vi "Move piezo slow.vi"(7 "error in (no error)":errorcluster, 8 "MOVE TO [MICRON]":dbl=1.0 format="%0.2f", 9 "notifier out":refnum<notifier>, 10 "Cluster":T1={"physical channels"="Dev5/ao0", "MAX   VOLTAGE"=10.0, "MIN   VOLTAGE"=0.0}) -> (0 "error out":errorcluster, 3 "Cluster 2":T1={"physical channels"="Dev5/ao0", "MAX   VOLTAGE"=10.0, "MIN   VOLTAGE"=0.0})   [LabVIEW 2013]
uses:
  Piezo/Piezo display.ctl
  Untitled Project 3 Andrea/piezo new/Hardware Configuration Piezo out.ctl
  <vilib>/Analysis/1siggen.llb/Ramp Pattern by Samples.vi
  <vilib>/DAQmx/write.llb/DAQmx Write (Analog DBL 1Chan 1Samp).vi
  <vilib>/DAQmx/create/channels.llb/DAQmx Create Channel (AO-Voltage-Basic).vi
  <vilib>/DAQmx/miscellaneous.llb/DAQmx Fill In Error Info.vi
  <vilib>/Analysis/NI_AALBase.lvlib
  Piezo/Piezo.lvlib
panel:
  out "PiezoPosition":sgl
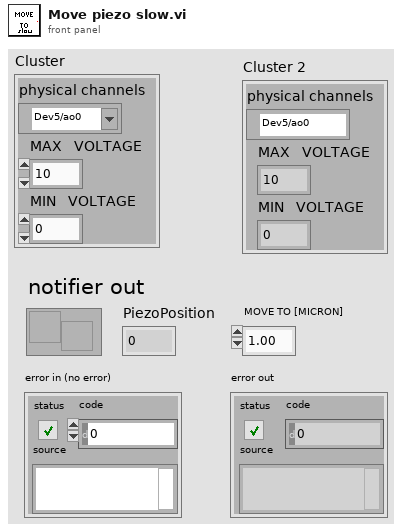
[diagram p1: front panel]
types:
  T1 = typedef "Hardware Configuration Piezo out.ctl" = cluster{"physical channels":tag, "MAX   VOLTAGE":dbl, "MIN   VOLTAGE":dbl}
  T2 = typedef "Piezo.lvlib/Piezo display.ctl" = cluster{"PiezoPosition":sgl, "Counter Time":i32}
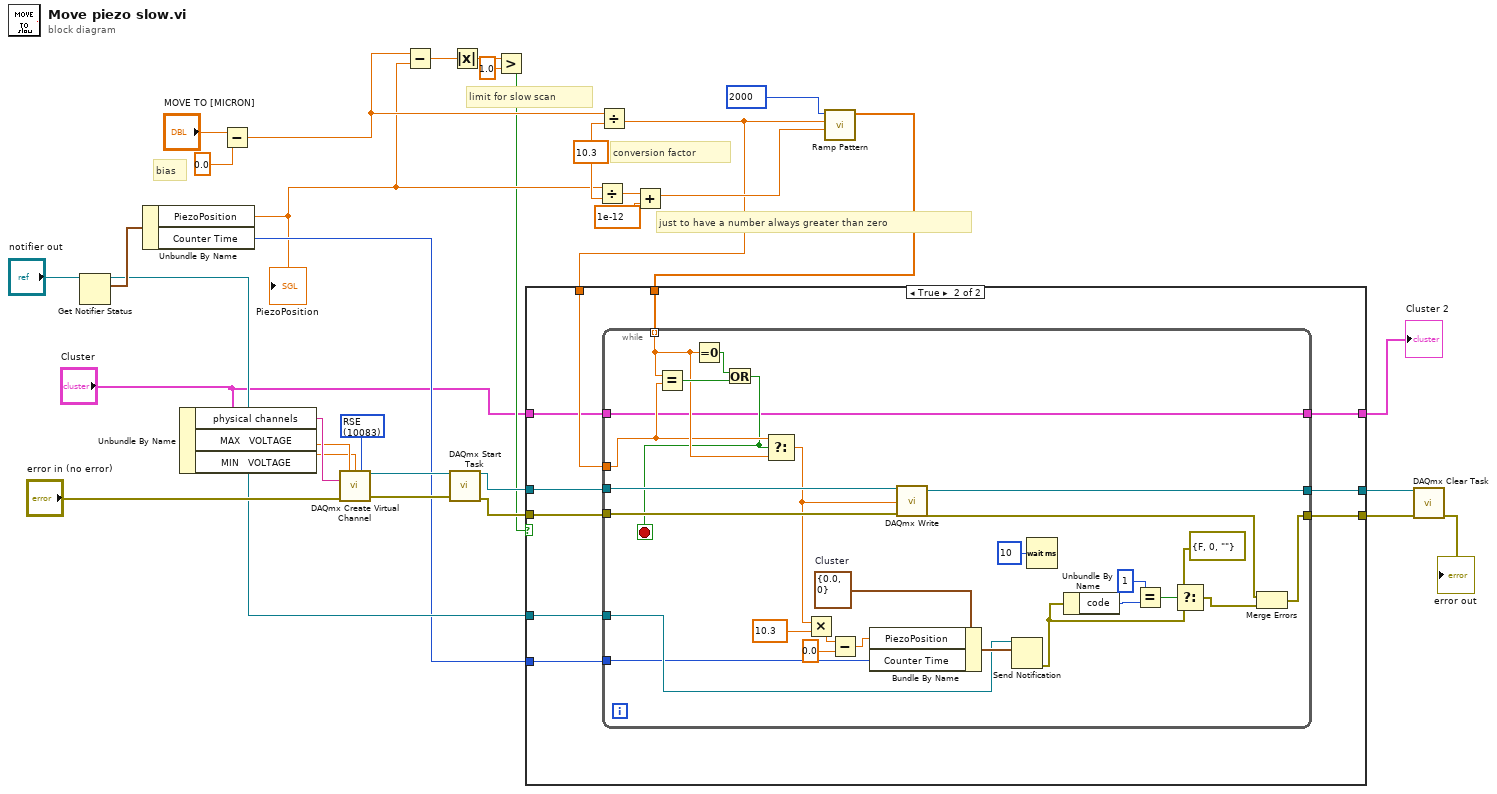
[diagram p0: block diagram]
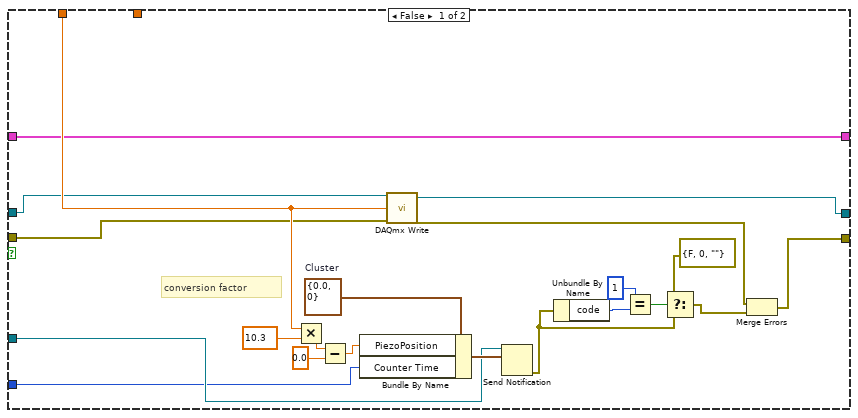
[diagram p2: hidden frame]
diagram:
  w25 = 10083 items=["Default"=-1, "RSE"=10083, "Differential"=10106, "Pseudodifferential"=12529] ("output terminal configuration")
  w30 = 10.3
  # "limit for slow scan"
  # "just to have a number always greater than zero"
  # "bias"
  # "conversion factor"
  n1 = Get Notifier Status(notifier="notifier out") -> (notifier out=w13:refnum<notifier>, current notification=w26:T2)  [unwired: 1 in, 3 out]
  n2 = Unbundle By Name(w26) -> ("PiezoPosition"=w4:sgl, "Counter Time"=w12:i32)
  "PiezoPosition" <- w4
  n3 = Unbundle By Name("Cluster") -> ("physical channels"=w22:tag, "MAX   VOLTAGE"=w21:dbl, "MIN   VOLTAGE"=w20:dbl)
  n4 = Subtract(x="MOVE TO [MICRON]", y=0.0) -> (x-y=w5:dbl)
  n5 = call-poly <vilib>:"DAQmx Create Virtual Channel.vi"("maximum value"=w21, "minimum value"=w20, "output terminal configuration"=w25, "physical channels"=w22, "error in"="error in (no error)") -> ("task out"=w24:refnum<k21>, "error out"=w23:errorcluster)  [unwired: 9 in]
  n6 = Subtract(x=w5, y=w4) -> (x-y=w8:dbl)
  n7 = call <vilib>:"DAQmx Start Task.vi"("task/channels in"=w24, "error in"=w23) -> ("task out"=w16:refnum<k21>, "error out"=w15:errorcluster)  [unwired: 12 in]
  n8 = Absolute Value(x=w8) -> (abs(x)=w7:dbl)
  n9 = Greater?(x=w7, y=1.0) -> (0:w3:bool)
  n10 = Divide(x=w4, y=w30) -> (x/y=w31:dbl)
  n11 = Divide(x=w5, y=w30) -> (x/y=w28:dbl)
  n12 = Add(x=w31, y=1e-12) -> (x+y=w32:dbl)
  n13 = call-poly <vilib>:"Ramp Pattern.vi"("start"=w32, "end"=w28, "samples"=2000) -> ("Ramp Pattern"=w29:dbl[])  [unwired: 7 in, 1 out]
  n14 = case shown="True" w3 {
    tunnel: w29 -> [_ w64]
    tunnel: w28 -> [w41 w63]
    tunnel: [w38 w62] -> w18
    tunnel: [w37 w61] -> w17
    tunnel: w16 -> [w40 w60]
    tunnel: w15 -> [w39 w59]
    tunnel: "Cluster" -> [w34 w58]
    tunnel: [w34 w57] -> w1
    tunnel: w13 -> [w36 w56]
    tunnel: w12 -> [w35 w55]
    frame False {
      w53 = T2 {"PiezoPosition"=0.0, "Counter Time"=0}  # Cluster
      # "conversion factor"
      n15 = Multiply(x=w41, y=10.3) -> (x*y=w43:dbl)
      n16 = Subtract(x=w43, y=0.0) -> (x-y=w44:dbl)
      n17 = Bundle By Name(cluster=w53, "PiezoPosition"=w44, "Counter Time"=w35) -> (w54:T2)
      n18 = call-poly <vilib>:"DAQmx Write.vi"("task/channels in"=w40, "data"=w41, "error in"=w39) -> ("task out"=w38:refnum<k21>, "error out"=w48:errorcluster)  [unwired: 10 in, 1 out]
      n19 = Send Notification(notification=w54, notifier=w36) -> (error out=w47:errorcluster)  [unwired: 1 in, 1 out]
      n20 = Unbundle By Name(w47) -> ("code"=w52:i32)
      n21 = Equal?(x=1, y=w52) -> (x = y?=w50:bool)
      n22 = Select(t=errorcluster {"status"=FALSE, "code"=0, "source"=""} ("error constant"), s=w50, f=w47) -> (s? t:f=w46:errorcluster)
      n23 = Merge Errors(w48, w46) -> (w37:errorcluster)
    }
    frame True {
      n24 = while {
        tunnel: w60 -> [w91]
        tunnel: w59 -> [w90]
        tunnel: [w89] -> w62
        tunnel: [w70] -> w61
        tunnel: w64 -> [w86] mode=indexing
        tunnel: w63 -> [w85]
        tunnel: w58 -> [w82]
        tunnel: [w82] -> w57
        tunnel: w56 -> [w80]
        tunnel: w55 -> [w78]
        stop <- w84 stop-if-true
        w79 = T2 {"PiezoPosition"=0.0, "Counter Time"=0}  # Cluster
        n25 = Equal?(x=w86, y=w85) -> (x = y?=w87:bool)
        n26 = Equal To 0?(x=w86) -> (x = 0?=w88:bool)
        n27 = Or(x=w88, y=w87) -> (x .or. y?=w84:bool)
        n28 = Select(t=w85, s=w84, f=w86) -> (s? t:f=w68:dbl)
        n29 = Multiply(x=w68, y=10.3) -> (x*y=w66:dbl)
        n30 = Subtract(x=w66, y=0.0) -> (x-y=w67:dbl)
        n31 = Bundle By Name(cluster=w79, "PiezoPosition"=w67, "Counter Time"=w78) -> (w81:T2)
        n32 = call-poly <vilib>:"DAQmx Write.vi"("task/channels in"=w91, "data"=w68, "error in"=w90) -> ("task out"=w89:refnum<k21>, "error out"=w73:errorcluster)  [unwired: 10 in, 1 out]
        n33 = Send Notification(notification=w81, notifier=w80) -> (error out=w72:errorcluster)  [unwired: 1 in, 1 out]
        n34 = Wait (ms)(milliseconds to wait=u32 10) -> ()  [unwired: 1 out]
        n35 = Unbundle By Name(w72) -> ("code"=w77:i32)
        n36 = Equal?(x=1, y=w77) -> (x = y?=w75:bool)
        n37 = Select(t=errorcluster {"status"=FALSE, "code"=0, "source"=""} ("error constant"), s=w75, f=w72) -> (s? t:f=w71:errorcluster)
        n38 = Merge Errors(w73, w71) -> (w70:errorcluster)
      }
    }
  }
  "Cluster 2" <- w1
  n39 = call <vilib>:"DAQmx Clear Task.vi"("task in"=w18, "error in"=w17) -> ("error out"=→"error out":errorcluster)  [unwired: 13 in]
